vi "Query File List Status.vi"(0 "VISA resource name":refnum<visa-resource-name>, 5 "List File Type  (0:Hard Copy)":i32(ring) items=["Hard Copy", "Parameter", "System Info", "Trace"], 7 "Application (0:Spectrum Analyzer)":i32(ring) items=["Spectrum Analyzer", "Phase Noise"], 9 "Driver Letter (D)":string="D", 11 "error in (no error)":errorcluster) -> (4 "VISA resource name out":refnum<visa-resource-name>, 6 "Number of Files":i32, 8 "Files":string[](array[string]), 15 "error out":errorcluster)   [LabVIEW 2020, in "Anritsu Signal Analyzer Series.lvlib"]
doc: "Queries the file list status."
uses:
  Anritsu Signal Analyzer Series.lvlib
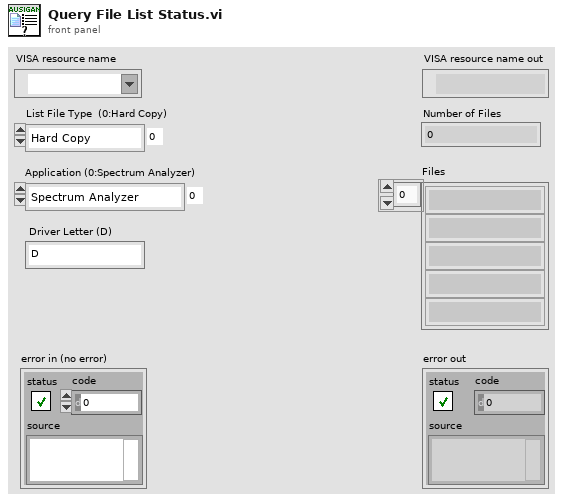
[diagram p1: front panel]
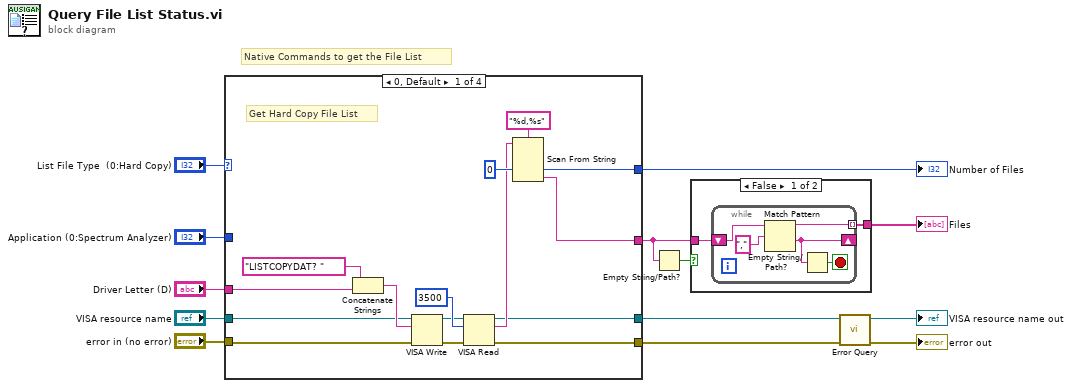
[diagram p0: block diagram]
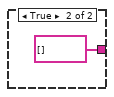
[diagram p2: hidden frame]
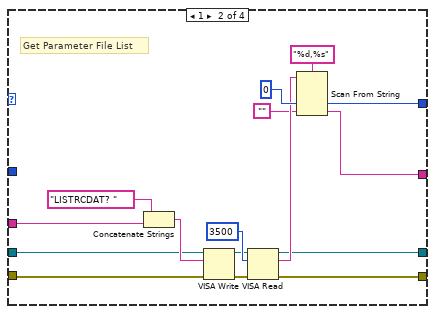
[diagram p3: hidden frame]
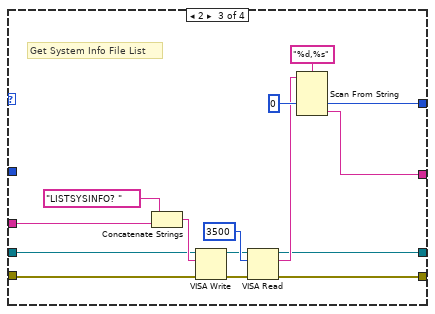
[diagram p4: hidden frame]
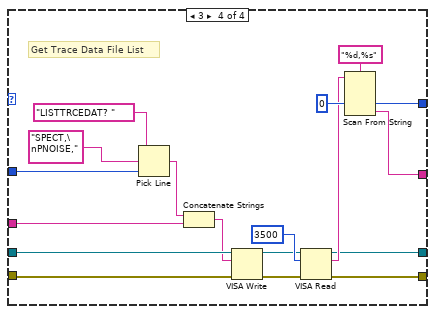
[diagram p5: hidden frame]
diagram:
  # "Native Commands to get the File List"
  n1 = case shown="0, Default" "List File Type  (0:Hard Copy)" {
    tunnel: "Driver Letter (D)" -> [w21 w37 w52 w65]
    tunnel: [w15 w31 w46 w67] -> w9
    tunnel: "Application (0:Spectrum Analyzer)" -> [_ _ _ w61]
    tunnel: "VISA resource name" -> [w20 w36 w51 w72]
    tunnel: "error in (no error)" -> [w19 w35 w50 w71]
    tunnel: [w18 w34 w49 w70] -> w4
    tunnel: [w17 w33 w48 w69] -> w3
    tunnel: [w14 w30 w45 w66] -> w1
    frame 0, Default {
      # "Get Hard Copy File List"
      n2 = Concatenate Strings("LISTCOPYDAT? " ("_Command"), w21) -> (w27:string)
      n3 = VISA Write(VISA resource name=w20, write buffer=w27, error in (no error)=w19) -> (VISA resource name out=w22:refnum<visa-resource-name>, error out=w16:errorcluster)  [unwired: 1 out]
      n4 = VISA Read(VISA resource name=w22, byte count=u32 3500 ("byte count (0)"), error in (no error)=w16) -> (VISA resource name out=w18:refnum<visa-resource-name>, read buffer=w24:string, error out=w17:errorcluster)  [unwired: 1 out]
      n5 = Scan From String(format string="%d,%s" ("Format String"), input string=w24, default 1=0 ("_Default")) -> (output 1=w15:i32, output 2=w14:string)  [unwired: 3 in, 3 out]
    }
    frame 1 {
      # "Get Parameter File List"
      n6 = Concatenate Strings("LISTRCDAT? " ("_Command"), w37) -> (w43:string)
      n7 = VISA Write(VISA resource name=w36, write buffer=w43, error in (no error)=w35) -> (VISA resource name out=w38:refnum<visa-resource-name>, error out=w32:errorcluster)  [unwired: 1 out]
      n8 = VISA Read(VISA resource name=w38, byte count=u32 3500 ("byte count (0)"), error in (no error)=w32) -> (VISA resource name out=w34:refnum<visa-resource-name>, read buffer=w40:string, error out=w33:errorcluster)  [unwired: 1 out]
      n9 = Scan From String(format string="%d,%s" ("Format String"), input string=w40, default 1=0 ("_Default"), default 2="") -> (output 1=w31:i32, output 2=w30:string)  [unwired: 2 in, 3 out]
    }
    frame 2 {
      # "Get System Info File List"
      n10 = Concatenate Strings("LISTSYSINFO? " ("_Command"), w52) -> (w58:string)
      n11 = VISA Write(VISA resource name=w51, write buffer=w58, error in (no error)=w50) -> (VISA resource name out=w53:refnum<visa-resource-name>, error out=w47:errorcluster)  [unwired: 1 out]
      n12 = VISA Read(VISA resource name=w53, byte count=u32 3500 ("byte count (0)"), error in (no error)=w47) -> (VISA resource name out=w49:refnum<visa-resource-name>, read buffer=w55:string, error out=w48:errorcluster)  [unwired: 1 out]
      n13 = Scan From String(format string="%d,%s" ("Format String"), input string=w55, default 1=0 ("_Default")) -> (output 1=w46:i32, output 2=w45:string)  [unwired: 3 in, 3 out]
    }
    frame 3 {
      # "Get Trace Data File List"
      n14 = Pick Line(string ("")="LISTTRCEDAT? " ("_Command"), multi-line string="SPECT,\nPNOISE," ("string"), line index=w61) -> (output string=w60:string)
      n15 = Concatenate Strings(w60, w65) -> (w64:string)
      n16 = VISA Write(VISA resource name=w72, write buffer=w64, error in (no error)=w71) -> (VISA resource name out=w73:refnum<visa-resource-name>, error out=w68:errorcluster)  [unwired: 1 out]
      n17 = VISA Read(VISA resource name=w73, byte count=u32 3500 ("byte count (0)"), error in (no error)=w68) -> (VISA resource name out=w70:refnum<visa-resource-name>, read buffer=w75:string, error out=w69:errorcluster)  [unwired: 1 out]
      n18 = Scan From String(format string="%d,%s" ("Format String"), input string=w75, default 1=0 ("_Default")) -> (output 1=w67:i32, output 2=w66:string)  [unwired: 3 in, 3 out]
    }
  }
  "Number of Files" <- w9
  n19 = Empty String/Path?(string/path=w1) -> (empty?=w2:bool)
  n20 = case shown="False" w2 {
    tunnel: [w79 string[] []] -> w6
    tunnel: w1 -> [w78 _]
    frame False {
      n21 = while {
        shift-right: [w80] -> _
        shift-left: w78 -> [w82]
        tunnel: [w83] -> w79 mode=indexing
        stop <- w81 stop-if-true
        n22 = Match Pattern(string=w82, regular expression=",") -> (before substring=w83:string, after substring=w80:string)  [unwired: 1 in, 2 out]
        n23 = Empty String/Path?(string/path=w80) -> (empty?=w81:bool)
      }
    }
    frame True {
    }
  }
  "Files" <- w6
  n24 = call "Error Query.vi"("error in (no error)"=w3, "VISA resource name"=w4) -> ("error out"=→"error out":errorcluster, "VISA resource name out"=→"VISA resource name out":refnum<visa-resource-name>)  [unwired: 6 in, 2 out]
